vi "Digital Out Test_v1.vi"() -> (0 "error out":errorcluster, 3 "Pass?":bool)   [LabVIEW 2022 SP3]
panel:
  out "Instructional Msg":string
  in  "OK Button":bool
  in  "bypass":bool
  in  "stop":bool
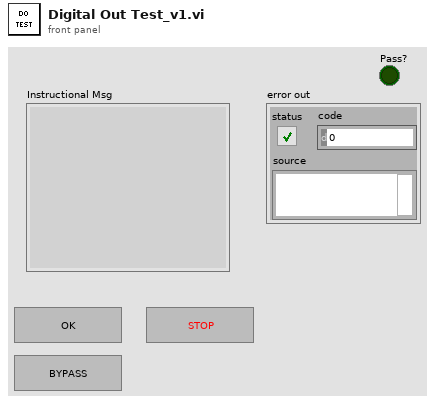
[diagram p1: front panel]
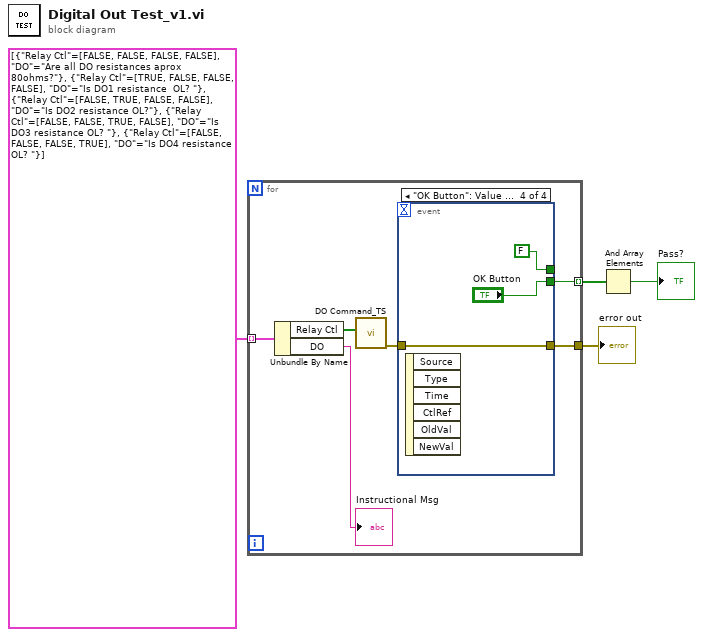
[diagram p0: block diagram]
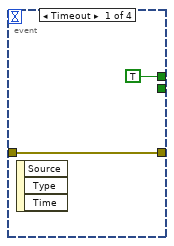
[diagram p2: hidden frame]
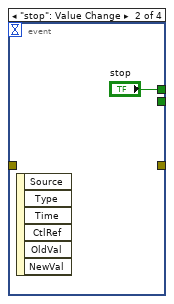
[diagram p3: hidden frame]
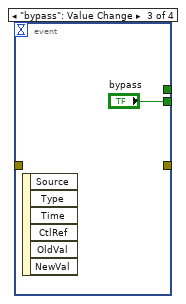
[diagram p4: hidden frame]
diagram:
  n1 = for {
    tunnel: cluster{"Relay Ctl":bool[], "DO":string}[] [{"Relay Ctl"=[FALSE, FALSE, FALSE, FALSE], "DO"="Are all DO resistances aprox 80ohms?"}, {"Relay Ctl"=[TRUE, FALSE, FALSE, FALSE], "DO"="Is DO1 resistance  OL? "}, {"Relay Ctl"=[FALSE, TRUE, FALSE, FALSE], "DO"="Is DO2 resistance OL?"}, {"Relay Ctl"=[FALSE, FALSE, TRUE, FALSE], "DO"="Is DO3 resistance OL? "}, {"Relay Ctl"=[FALSE, FALSE, FALSE, TRUE], "DO"="Is DO4 resistance OL? "}] -> [w10] mode=indexing
    tunnel: [w6] -> w3 mode=indexing
    tunnel: [w5] -> w1
    n2 = Unbundle By Name(w10) -> ("Relay Ctl"=w9:bool[], "DO"=→"Instructional Msg":string)
    n3 = call "DO Command_TS.vi"("DO Command"=w9) -> ("error out"=w7:errorcluster)  [unwired: 9 in, 1 out]
    n4 = event shown="[3] \"OK Button\": Value Change" {
      selector: _ -> [_ _ _ _]
      dyn-events: _ -> [_ _ _ _]
      timeout: _ -> [_ _ _ _]
      tunnel: w7 -> [w12 _ _ w17]
      tunnel: [w12 _ _ w17] -> w5
      tunnel: [TRUE "stop" _ FALSE] -> _
      tunnel: [_ _ "bypass" "OK Button"] -> w6
      event Timeout {
        n5 = event-data() -> ()  [unwired: 1 in, 3 out]
      }
      event "stop": Value Change {
        n6 = event-data() -> ()  [unwired: 1 in, 6 out]
      }
      event "bypass": Value Change {
        n7 = event-data() -> ()  [unwired: 1 in, 6 out]
      }
      event "OK Button": Value Change {
        n8 = event-data() -> ()  [unwired: 1 in, 6 out]
      }
    }
  }
  "error out" <- w1
  n9 = And Array Elements(Boolean array=w3) -> (logical AND=→"Pass?":bool)
